vi "ASK пример.vi"() -> ()   [LabVIEW 2017]
uses:
  <vilib>/addons/Modulation/Digital/Channel Coding/MT Convolutional Encoder (Rate).vi
  <vilib>/addons/Modulation/Digital/Support/Common/Validators/mod_Validate Bit Stream.vi
  <vilib>/addons/Modulation/Digital/Channel Coding/Convolutional codes/mod_Convolutional encoder.vi
  <vilib>/addons/Modulation/Analog/support/mod_Set Error Source.vi
  <vilib>/addons/Modulation/Digital/Channel Coding/Convolutional codes/subVIs/mod_Generate encoder tap connections.vi
  <vilib>/addons/Modulation/Digital/Channel Coding/Convolutional codes/subVIs/mod_Perform convolutional encoding.vi
  <vilib>/addons/Modulation/Digital/Channel Coding/Block codes/subVIs/mod_Buffer block code info (I8).vi
  <vilib>/addons/Modulation/Digital/Channel Coding/Convolutional codes/subVIs/mod_Generate valid reset (convolutional, I8).vi
  <vilib>/addons/Modulation/Digital/General/MT Generate ASK system parameters (M).vi
  <vilib>/addons/Modulation/Digital/Support/Common/Validators/mod_Generate Filter Coefficients Validate.vi
  <vilib>/addons/Modulation/Digital/General/subVIs/mod_Generate Filter Coefficients.vi
  <vilib>/addons/Modulation/Digital/Channel Coding/Convolutional codes/subVIs/mod_Select known generator matrix.vi
  <vilib>/addons/Modulation/Digital/Support/Common/Validators/mod_Validate Convolutional Encoder prms.vi
  <vilib>/addons/Modulation/Analog/MT Upconvert Baseband (Real).vi
  <vilib>/addons/Modulation/Analog/MT Downconvert Passband (Real).vi
  <vilib>/addons/Modulation/Digital/Channel Coding/MT Convolutional Decoder (Viterbi Hard Decision, Rate).vi
  <vilib>/Waveform/DWDTOps.llb/DWDT Analog to Digital.vi
  <vilib>/addons/Modulation/niDMT.lvlib
  <vilib>/addons/Modulation/niAMT.lvlib
panel:
  out "Массив с":dbl[](array[numeric])
  out "Вырезка из массива 2":dbl[](array[numeric])
  out "Digital Waveform Graph 4":digitalwaveform(graph)
  out "Digital Waveform Graph 3":digitalwaveform(graph)
  in  "constraint length (K)":i32=3
  in  "rate (k/n)":enum16{"1/2", "1/3", "1/4", "2/3", "3/4"}(ring)
  out "Массив выход":dbl[](array[numeric])
  out "Waveform Graph 2":cluster{"t0":dbl, "dt":dbl, "Y":dbl[]}(graph)
  in  "Сколько битов брать":i32=4
  out "Массив с паузами":dbl[](array[numeric])
  in  "Количество бит":i32=8
  out "Вырезка из массива":dbl[](array[numeric])
  out "Биты на выходе 1":dbl[](array[numeric])
  out "Digital Waveform Graph":digitalwaveform(graph)
  in  "pulse shaping filter (none) 2":T1(ring) caption="pulse shaping filter (none)"
  in  "passband bandwidth (Hz)":dbl format="%.2p"
  in  "carrier frequency (Hz) 2":dbl caption="carrier frequency (Hz)" min=-0.5 max=0.5 format="%.2p"
  out "Waveform Graph":waveform(dbl)[](graph)
  out "Rs":dbl
  in  "carrier frequency (Hz)":dbl min=-0.5 max=0.5 format="%.2f"
  in  "pulse shaping filter (none)":T1(ring)
  in  "Ts":dbl
  in  "Fs":dbl
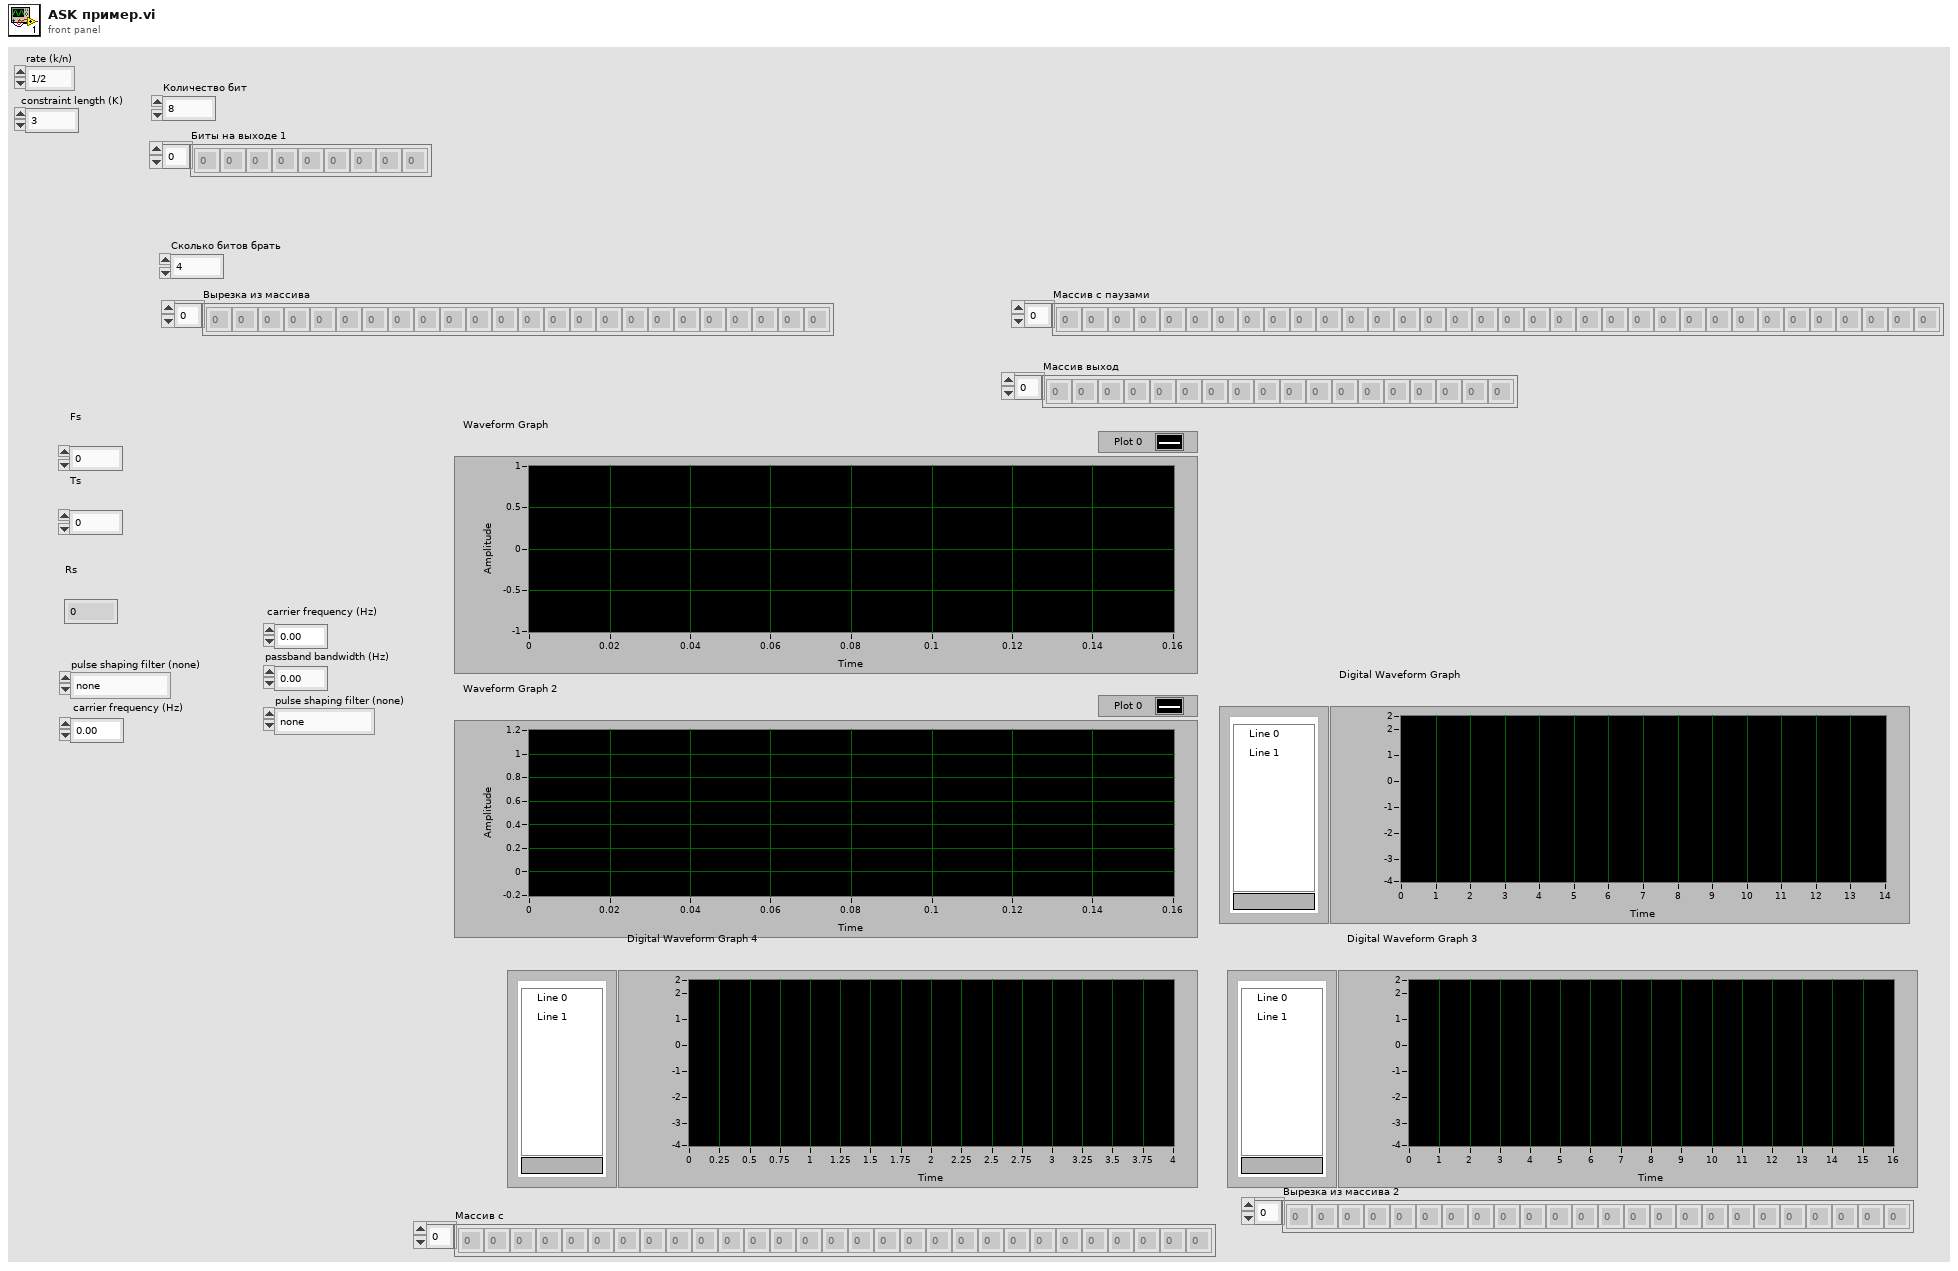
[diagram p1: front panel]
types:
  T1 = enum16{"none", "Raised Cosine", "Root Raised Cos", "Gaussian"}
  T2 = enum16{"FSK", "PSK", "QAM", "MSK", "PAM", "ASK", "CPM"}
  T3 = cluster{"samples per symbol (16)":i32, "symbol map":cdb[]}
  T4 = typedef "niAMT.lvlib/Complex Data Waveform.ctl" = cluster{"t0":dbl, "dt":dbl, "Y":cdb[]}
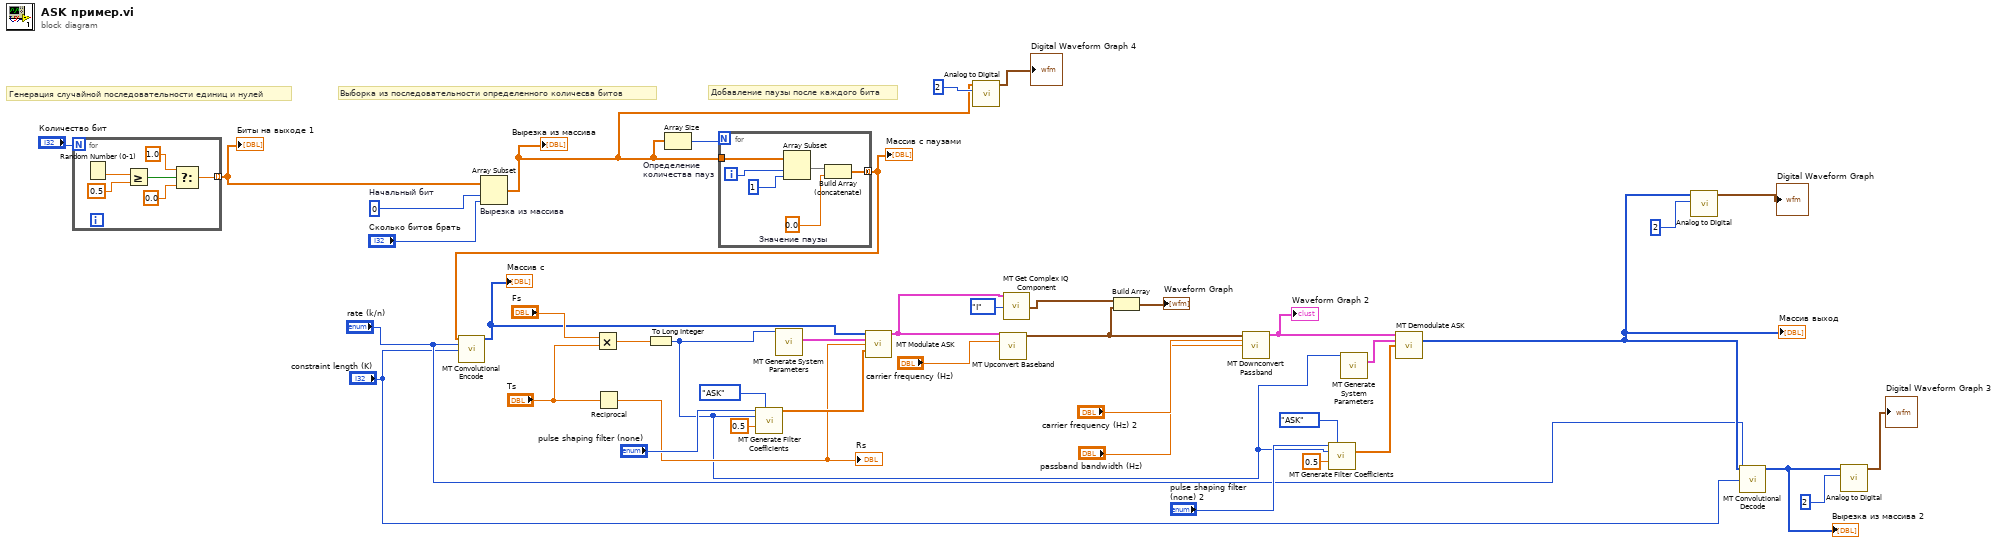
[diagram p0: block diagram]
diagram:
  w18 = 0  # Начальный бит
  # "Добавление паузы после каждого бита"
  # "Выборка из последовательности определенного количесва битов"
  # "Генерация случайной последовательности единиц и нулей"
  n1 = for {
    N: "Количество бит" -> [_]
    tunnel: [w43] -> w16 mode=indexing
    n2 = Random Number (0-1)() -> (number: 0 to 1=w48:dbl)
    n3 = Greater Or Equal?(x=w48, y=0.5) -> (x >= y?=w46:bool)
    n4 = Select(t=1.0, s=w46, f=0.0) -> (s? t:f=w43:dbl)
  }
  "Биты на выходе 1" <- w16
  n5 = Array Subset "Вырезка из массива"(array=w16, index=w18, length="Сколько битов брать") -> (w3:dbl[])
  "Вырезка из массива" <- w3
  n6 = Multiply(x="Fs", y="Ts") -> (x*y=w40:dbl)
  n7 = Reciprocal(x="Ts") -> (1/x=w31:dbl)
  "Rs" <- w31
  n8 = To Long Integer(number=w40) -> (32bit integer=w12:i32)
  n9 = Array Size "Определение количества пауз"(array=w3) -> (size(s)=w15:i32)
  n10 = for {
    N: w15 -> [_]
    tunnel: w3 -> [w51]
    tunnel: [w50] -> w11 mode=concatenating
    i -> [w49]
    w52 = 0.0  # Значение паузы
    n11 = Array Subset(array=w51, index=w49, length=1) -> (w53:dbl[])
    n12 = Build Array (concatenate)(w53, w52) -> (w50:dbl[])
  }
  "Массив с паузами" <- w11
  n13 = call-poly <vilib>:"MT Convolutional Encode.vi"("input bit stream"=w11, "rate (k/n)"="rate (k/n)", "constraint length (K)"="constraint length (K)") -> ("output bit stream"=w1:i8[])  [unwired: 10 in, 2 out]
  "Массив с" <- w1
  n14 = call <vilib>:"MT Generate Filter Coefficients.vi"("pulse shaping filter (none)"="pulse shaping filter (none)", "modulation type"=T2."ASK", "pulse shaping samples per symbol (16)"=w12, "filter parameter"=0.5) -> ("pulse shaping filter coefficients"=w37:dbl[])  [unwired: 9 in, 2 out]
  n15 = call-poly <vilib>:"MT Generate System Parameters.vi"("samples per symbol (16)"=w12) -> ("ASK system parameters"=w36:T3)  [unwired: 12 in, 2 out]
  n16 = call <vilib>:"MT Modulate ASK.vi"("input bit stream"=w1, "ASK system parameters"=w36, "symbol rate (Hz)"=w31, "pulse shaping filter coefficients"=w37) -> ("output complex waveform"=w34:T4)  [unwired: 9 in, 2 out]
  n17 = call-poly <vilib>:"Analog to Digital.vi"("resolution (16 bit)"=2, "analog waveform"=w3) -> ("digital waveform"=→"Digital Waveform Graph 4":digitalwaveform)  [unwired: 6 in, 3 out]
  n18 = call-poly <vilib>:"MT Upconvert Baseband.vi"("baseband waveform (complex)"=w34, "carrier frequency (Hz)"="carrier frequency (Hz)") -> ("passband waveform"=w28:waveform(dbl))  [unwired: 12 in, 1 out]
  n19 = call <vilib>:"MT Get Complex IQ Component.vi"("IQ data (complex) in"=w34, "component choice"=enum16{"I", "Q", "Magnitude", "Phase"}."I") -> ("CE component"=w30:waveform(dbl))  [unwired: 11 in, 2 out]
  n20 = Build Array(w30, w28) -> (→"Waveform Graph":waveform(dbl)[])
  n21 = call-poly <vilib>:"MT Downconvert Passband.vi"("Waveform"=w28, "carrier frequency (Hz)"="carrier frequency (Hz) 2", "passband bandwidth (Hz)"="passband bandwidth (Hz)") -> ("downconverted waveform (complex baseband)"=w14:T4)  [unwired: 9 in, 3 out]
  "Waveform Graph 2" <- w14
  n22 = call <vilib>:"MT Generate Filter Coefficients.vi"("pulse shaping filter (none)"="pulse shaping filter (none) 2", "modulation type"=T2."ASK", "pulse shaping samples per symbol (16)"=w12, "filter parameter"=0.5) -> ("matched filter coefficients"=w23:dbl[])  [unwired: 9 in, 2 out]
  n23 = call-poly <vilib>:"MT Generate System Parameters.vi"("samples per symbol (16)"=w12) -> ("ASK system parameters"=w13:T3)  [unwired: 12 in, 2 out]
  n24 = call <vilib>:"MT Demodulate ASK.vi"("input complex waveform"=w14, "ASK system parameters"=w13, "matched filter coefficients"=w23) -> ("output bit stream"=w10:i8[])  [unwired: 8 in, 4 out]
  "Массив выход" <- w10
  n25 = call-poly <vilib>:"Analog to Digital.vi"("resolution (16 bit)"=2, "analog waveform"=w10) -> ("digital waveform"=→"Digital Waveform Graph":digitalwaveform)  [unwired: 6 in, 3 out]
  n26 = call-poly <vilib>:"MT Convolutional Decode.vi"("input bit stream"=w10, "rate (k/n)"="rate (k/n)", "constraint length (K)"="constraint length (K)") -> ("output bit stream"=w2:i8[])  [unwired: 10 in, 2 out]
  "Вырезка из массива 2" <- w2
  n27 = call-poly <vilib>:"Analog to Digital.vi"("resolution (16 bit)"=2, "analog waveform"=w2) -> ("digital waveform"=→"Digital Waveform Graph 3":digitalwaveform)  [unwired: 6 in, 3 out]
